vi "FilterArrayAndIndexOutput.vi"() -> ()   [LabVIEW 2019]
panel:
  out "Array":i32[](array[numeric])
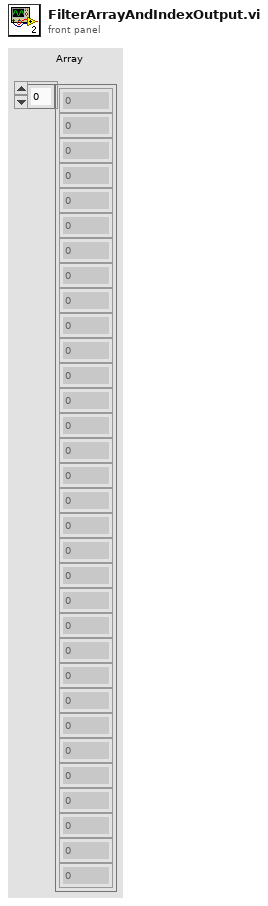
[diagram p1: front panel]
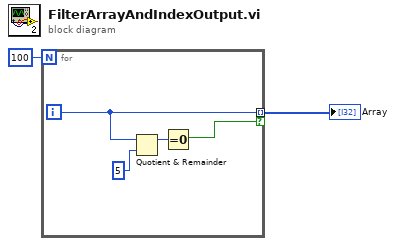
[diagram p0: block diagram]
diagram:
  n1 = for {
    N: 100 -> [_]
    tunnel: [w6] -> w1 mode=indexing if=w3
    i -> [w6]
    n2 = Quotient & Remainder(x=w6, y=5) -> (x-y*floor(x/y)=w4:i32)  [unwired: 1 out]
    n3 = Equal To 0?(x=w4) -> (x = 0?=w3:bool)
  }
  "Array" <- w1
